vi "Set Measurement Name.vi"(8 "error in (no error)":errorcluster, 11 "Servo MSMT in":refnum<class "Servo MSMT.lvclass">) -> (0 "error out":errorcluster, 3 "Servo MSMT out":refnum<class "Servo MSMT.lvclass">)   [LabVIEW 2018, in "Servo MSMT.lvlib" / "Servo MSMT.lvclass"]
uses:
  Servo MSMT.lvclass
  C:/Sequence Automation/Plugins/Measurement Interface.lvlibp/Measurement Interface.lvclass
  Plugins/Measurement Interface.lvlibp/Private Methods/Measurement Parameters/Read Measurement Parameters.vi
  Plugins/Measurement Interface.lvlibp/Private Methods/Measurement Name/Read Measurement Name.vi
  Plugins/Measurement Interface.lvlibp/Private Methods/Test Group Manager/Read Test Group Manager.vi
  Plugins/Measurement Interface.lvlibp/Private Methods/Test Group Manager/Write Test Group Manager.vi
  Plugins/Measurement Interface.lvlibp/Private Methods/Measurement Name/Write Measurement Name.vi
  Plugins/String Database.lvlibp/String Database.lvclass
  Plugins/Test Group Manager.lvlibp/Test Group Manager.lvclass
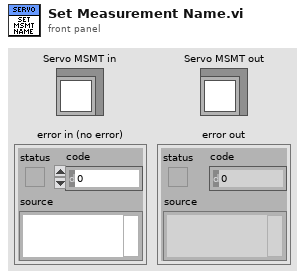
[diagram p1: front panel]
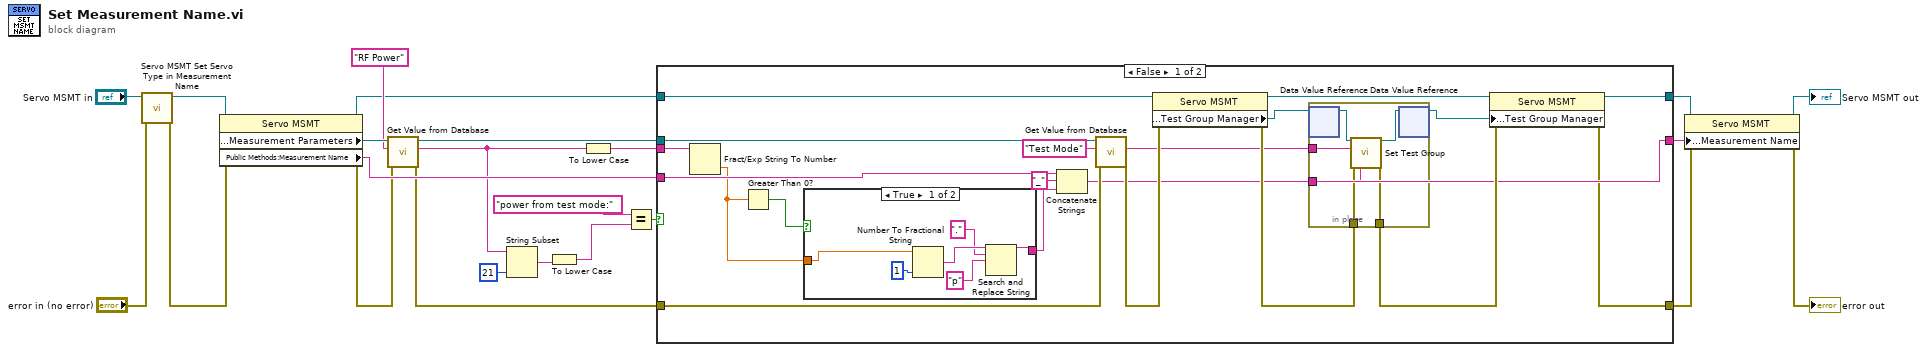
[diagram p0: block diagram]
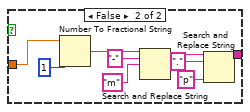
[diagram p2: hidden frame]
diagram:
  n1 = call-dynamic "Servo MSMT Set Servo Type in Measurement Name.vi"("error in (no error)"="error in (no error)", "Servo MSMT in"="Servo MSMT in") -> ("error out"=w16:errorcluster, "Servo MSMT out"=w15:refnum<class "Servo MSMT.lvclass">)  [unwired: 8 in]
  n2 = property class="Servo MSMT"(reference=w15, error in=w16) -> (reference out=w10:refnum<class "Servo MSMT.lvclass">, error out=w14:errorcluster, "Protected Methods:Measurement Parameters"=w22:refnum<class "String Database.lvclass">, "Public Methods:Measurement Name"=w20:string)
  n3 = call "Get Value from Database.vi"("error in (no error)"=w14, "Entry Name"="RF Power", "Message in"=w22) -> ("error out"=w3:errorcluster, "Entry Value"=w9:string, "Message out"=w1:refnum<class "String Database.lvclass">)  [unwired: 5 in, 1 out]
  n4 = String Subset(string=w9, length (rest)=21 ("length (rest)")) -> (substring=w7:string)  [unwired: 1 in]
  n5 = To Lower Case(string=w7) -> (all lower case string=w5:string)
  n6 = To Lower Case(string=w9) -> (all lower case string=w13:string)
  n7 = Equal?(x="power from test mode:" ("regular expression"), y=w5) -> (x = y?=w4:bool)
  n8 = case shown="False" w4 {
    tunnel: w20 -> [w43 w65]
    tunnel: [w31 w65] -> w17
    tunnel: [w27 w67] -> w11
    tunnel: w10 -> [w39 w67]
    tunnel: w13 -> [w42 _]
    tunnel: w3 -> [w35 w66]
    tunnel: [w29 w66] -> w2
    tunnel: w1 -> [w36 _]
    frame False {
      n9 = Fract/Exp String To Number(string=w42) -> (number=w40:dbl)  [unwired: 3 in, 1 out]
      n10 = Greater Than 0?(x=w40) -> (x > 0?=w41:bool)
      n11 = case shown="True" w41 {
        tunnel: [w50 w56] -> w25
        tunnel: w40 -> [w51 w57]
        frame True {
          n12 = Number To Fractional String(number=w51, precision (6)=i16 1 ("width (-)")) -> (F-format string=w54:string)  [unwired: 2 in]
          n13 = Search and Replace String(input string=w54, search string=".", replace string="p" ("replace string (\"\")")) -> (result string=w50:string)  [unwired: 5 in, 3 out]
        }
        frame False {
          n14 = Number To Fractional String(number=w57, precision (6)=i16 1) -> (F-format string=w64:string)  [unwired: 2 in]
          n15 = Search and Replace String(input string=w64, search string="-", replace string="m" ("replace string (\"\")")) -> (result string=w60:string)  [unwired: 5 in, 3 out]
          n16 = Search and Replace String(input string=w60, search string=".", replace string="p" ("replace string (\"\")")) -> (result string=w56:string)  [unwired: 5 in, 3 out]
        }
      }
      n17 = Concatenate Strings(w43, "_" ("string"), w25) -> (w31:string)
      n18 = call "Get Value from Database.vi"("error in (no error)"=w35, "Entry Name"="Test Mode", "Message in"=w36) -> ("error out"=w34:errorcluster, "Entry Value"=w32:string)  [unwired: 5 in, 2 out]
      n19 = property class="Servo MSMT"(reference=w39, error in=w34) -> (reference out=w28:refnum<class "Servo MSMT.lvclass">, error out=w38:errorcluster, "Protected Methods:Test Group Manager"=w30:refnum<data-value>)
      n20 = in-place {
        in-place-border: w38 -> [w49]
        in-place-border: [w48] -> w37
        in-place-border: w32 -> [w47]
        in-place-border: w31 -> [w46]
        n21 = in-place-dvr #1(w30) -> (w45:refnum<class "Test Group Manager.lvclass">)  [unwired: 1 out]
        n22 = call "Set Test Group.vi"("Test Group Manager in"=w45, "Test Group Name"=w47, "Input Power"=w46, "error in (no error)"=w49) -> ("Test Group Manager out"=w44:refnum<class "Test Group Manager.lvclass">, "error out"=w48:errorcluster)  [unwired: 14 in]
        n23 = in-place-dvr #1(w44) -> (w26:refnum<data-value>)  [unwired: 1 out]
      }
      n24 = property class="Servo MSMT"(reference=w28, error in=w37, "Protected Methods:Test Group Manager"=w26) -> (reference out=w27:refnum<class "Servo MSMT.lvclass">, error out=w29:errorcluster)
    }
    frame True, Default {
    }
  }
  n25 = property class="Servo MSMT"(reference=w11, error in=w2, "Public Methods:Measurement Name"=w17) -> (reference out=→"Servo MSMT out":refnum<class "Servo MSMT.lvclass">, error out=→"error out":errorcluster)
